vi "SubVI_initPidgeon.vi"   [LabVIEW 2017]
uses:
  <vilib>/Rock Robotics/WPI/ThirdParty/Phoenix-LabVIEW/Pigeon IMU/CTRE_PigeonIMU_TareType.ctl
  <vilib>/Rock Robotics/WPI/ThirdParty/Phoenix-LabVIEW/Pigeon IMU/CTRE_PigeonIMU_Open_CAN.vi
types:
  T1 = typedef "CTRE_PigeonIMU_TareType.ctl" = u8
  T2 = typedef "CTRE_PigeonIMU_DeviceRef.ctl" = cluster{"DeviceStatus":errorcluster, "Device Number":u8, "Type":T3, "Device ID":u32, "Handle":u64, "UsageFrame":u32, "Library Path":path}
  T3 = typedef "CTRE_PigeonIMU_ConnectionType.ctl" = u32
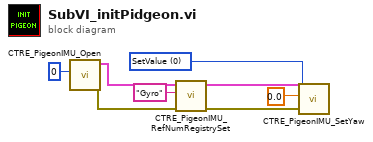
[diagram p0: block diagram]
diagram:
  w8 = T1 0 items=["SetValue"=0, "AddOffset"=1, "MatchCompass"=2, "SetOffset"=255] ("TareType (SetValue)")
  n1 = call-poly <vilib>:"CTRE_PigeonIMU_Open.vi"("Device Number"=u8 0) -> ("error out"=w3:errorcluster, "PigeonIMUDevRef"=w2:T2)  [unwired: 9 in]
  n2 = call <vilib>:"CTRE_PigeonIMU_RefNumRegistrySet.vi"("error in (no error)"=w3, "refnum name"="Gyro", "PigeonIMUDevRef"=w2) -> ("error out"=w6:errorcluster, "PigeonIMUDevRef"=w5:T2)  [unwired: 7 in]
  n3 = call <vilib>:"CTRE_PigeonIMU_SetYaw.vi"("error in (no error)"=w6, "TareType (SetValue)"=w8, "Value"=0.0, "PigeonIMUDevRef"=w5) -> ()  [unwired: 6 in, 2 out]
